vi "Max_&_Min_Array_2D.vi"(11 "Max & Min Array 2D":i8[][](array[numeric])=[[-3, 55, 41], [6, -1, 14], [-3, 2, -70], [-100, 1, 7]]) -> (0 "Indexs Min.":T1, 1 "Min. Value":i8, 2 "Indexs Max.":T1, 3 "Max. Value":i8)   [LabVIEW 2018]
uses:
  Controls/Rows_Columns.ctl
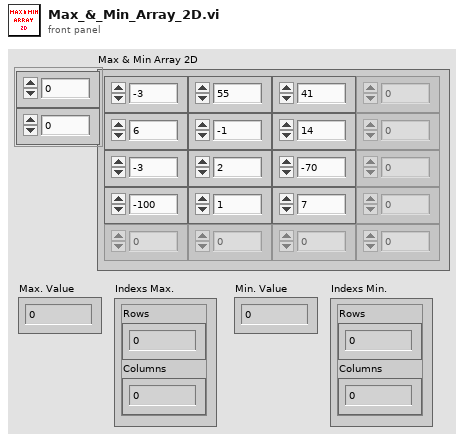
[diagram p1: front panel]
types:
  T1 = typedef "Rows_Columns.ctl" = cluster{"Rows":i32, "Columns":i32}
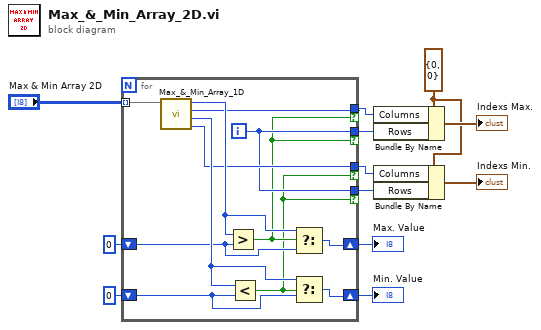
[diagram p0: block diagram]
diagram:
  w5 = T1 {"Rows"=0, "Columns"=0} ("Indexs Max.")
  n1 = for {
    tunnel: "Max & Min Array 2D" -> [w24] mode=indexing
    shift-right: [w16] -> w7
    shift-left: i8 0 -> [w20]
    shift-right: [w19] -> w6
    shift-left: i8 0 -> [w21]
    tunnel: [w18] -> w9 if=w14
    tunnel: [w17] -> w4 if=w13
    tunnel: [w15] -> w8 if=w14
    tunnel: [w15] -> w3 if=w13
    i -> [w15]
    n2 = call "Max_&_Min_Array_1D.vi"("Max & Min Array 1D"=w24) -> ("Index Min."=w17:i32, "Min. Value"=w22:i8, "Index Max."=w18:i32, "Max. Value"=w23:i8)  [unwired: 7 in]
    n3 = Greater?(x=w23, y=w20) -> (0:w14:bool)
    n4 = Less?(x=w22, y=w21) -> (x < y?=w13:bool)
    n5 = Select(t=w23, s=w14, f=w20) -> (s? t:f=w16:i8)
    n6 = Select(t=w22, s=w13, f=w21) -> (s? t:f=w19:i8)
  }
  "Max. Value" <- w7
  "Min. Value" <- w6
  n7 = Bundle By Name(cluster=w5, "Columns"=w9, "Rows"=w8) -> (→"Indexs Max.":T1)
  n8 = Bundle By Name(cluster=w5, "Columns"=w4, "Rows"=w3) -> (→"Indexs Min.":T1)
